vi "RT - Create Or Read Config.vi"(8 "error in":errorcluster) -> (0 "error out":errorcluster)   [LabVIEW 2018]
uses:
  Controls/Config.ctl
  Controls/Settings.ctl
  Controls/Parameters.ctl
  Controls/Timeouts.ctl
  Controls/ConfigString.ctl
  Controls/ConfigData.ctl
  Globals/Global - Configuration Options.vi
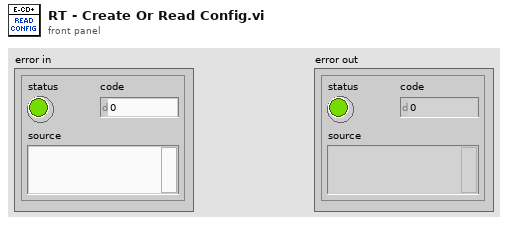
[diagram p1: front panel]
types:
  T1 = typedef "ConfigString.ctl" = cluster{"PDP (IN)":string[], "SETTINGS":string[], "TIMEOUTS (SEC)":string[]}
  T2 = typedef "Timeouts.ctl" = cluster{"TWTT Drive":dbl, "DL Drive":dbl, "DL Rotate":dbl, "BR Drive":dbl, "OT Engage":dbl, "PLUG Drive":dbl, "IT Engage":dbl, "IT 1REV":dbl, "IT nREV":dbl}
  T3 = typedef "Parameters.ctl" = cluster{"PDP (IN)":T4, "SETTINGS":T5, "TIMEOUTS (SEC)":T2}
  T4 = typedef "Config.ctl" = cluster{"TWTT OP":dbl, "TWTT PDP":dbl, "DLT OP":dbl, "DLT PDP 01":dbl, "DLT PDP 02":dbl, "BR OP":dbl, "BR TWT ALIGN":dbl, "BR DL ALIGN":dbl}
  T5 = typedef "Settings.ctl" = cluster{"HPL Low (PSI)":dbl, "HPL High (PSI)":dbl, "HPH Low (PSI)":dbl, "HPH High (PSI)":dbl, "AP Low (PSI)":dbl, "AP High (PSI)":dbl, "DL Clean (SEC)":dbl, "Reset (MIN)":dbl}
  T6 = typedef "ConfigData.ctl" = cluster{"PDP (IN)":dbl[], "SETTINGS":dbl[], "TIMEOUTS (SEC)":dbl[]}
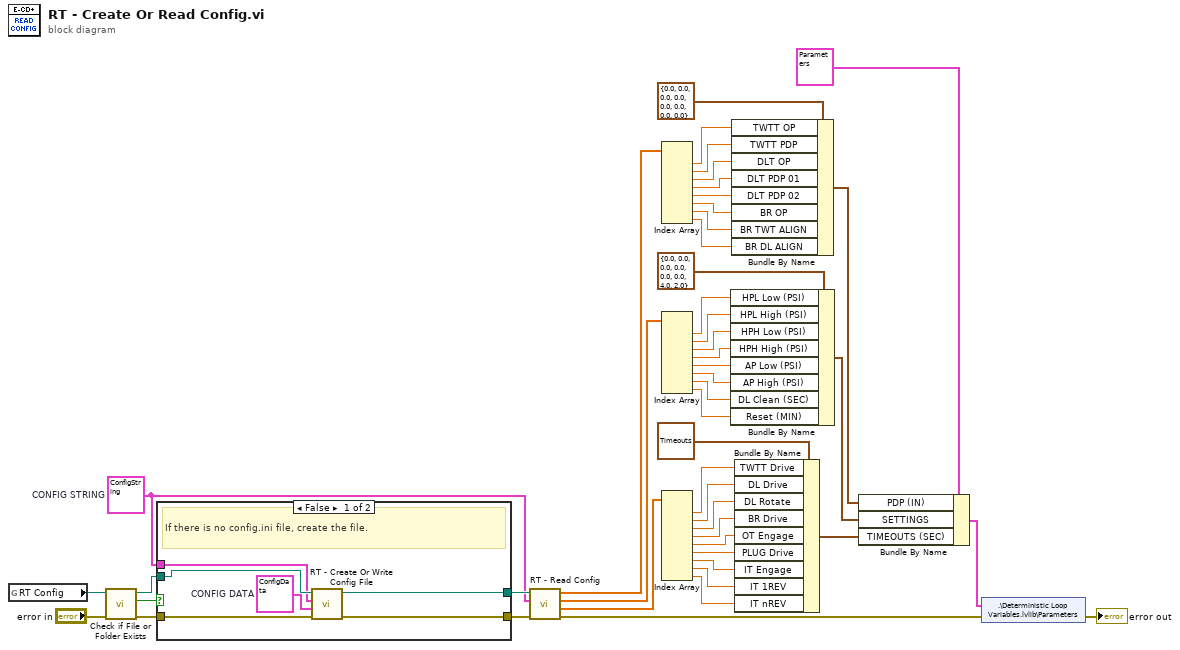
[diagram p0: block diagram]
diagram:
  w31 = T1 {"PDP (IN)"=["TWTT OP (IN)", "TWTT PDP (IN)", "DLT OP (IN)", "DLT PDP 01 (IN)", "DLT PDP 02 (IN)", "BR OP (IN)", "BR TWT ALIGN", "BR DL ALIGN (IN)"], "SETTINGS"=["HPL Low (PSI)", "HPL High (PSI)", "HPH Low (PSI)", "HPH High (PSI)", "AP Low (PSI)", "AP High (PSI)", "DL Clean (SEC)", "Reset (MIN)"], "TIMEOUTS (SEC)"=["TWTT Drive (SEC)", "DL Drive (SEC)", "DL Rotate (SEC)", "BR Drive (SEC)", "OT Engage (SEC)", "Plug Drive (SEC)", "IT Engage (SEC)", "IT 1REV (SEC)", "IT nREV (SEC)"]}  # CONFIG STRING
  n1 = global read "Global - Configuration Options.vi" "RT Config"() -> (w36:path)
  n2 = call <vilib>:"Check if File or Folder Exists.vi"("error in (no error)"="error in", "path"=w36) -> ("error out"=w35:errorcluster, "file or folder exists?"=w37:bool, "dup path"=w34:path)  [unwired: 7 in]
  n3 = case shown="False" w37 {
    tunnel: w35 -> [w52 w53]
    tunnel: w34 -> [w51 w54]
    tunnel: [w50 w53] -> w32
    tunnel: [w49 w54] -> w33
    tunnel: w31 -> [w48 _]
    frame False {
      w47 = T6 {"PDP (IN)"=[1.0, 2.2, 1.0, 1.744, 1.4, 5.3, 0.873, 8.975], "SETTINGS"=[100.0, 500.0, 200.0, 2800.0, 30.0, 180.0, 8.0, 2.0], "TIMEOUTS (SEC)"=[20.0, 20.0, 60.0, 20.0, 20.0, 60.0, 20.0, 30.0, 60.0]}  # CONFIG DATA
      # "If there is no config.ini file, create the file."
      n4 = call "RT - Create Or Write Config File.vi"("error in"=w52, "CONFIG DATA"=w47, "CONFIG STRING"=w48, "ConfigFile Path In"=w51) -> ("error out"=w50:errorcluster, "ConfigFile Path Out"=w49:path)  [unwired: 6 in]
    }
    frame True {
    }
  }
  n5 = call "RT - Read Config.vi"("error in"=w32, "CONFIG STRING"=w31, "ConfigFile Path In"=w33) -> ("error out"=w29:errorcluster, "TIMEOUTS (SEC)"=w15:dbl[], "SETTINGS"=w24:dbl[], "PDP (IN)"=w28:dbl[])  [unwired: 5 in]
  n6 = Index Array(array=w28) -> (element #1=w27:dbl, element #2=w26:dbl, element #3=w25:dbl, element #4=w5:dbl, element #5=w4:dbl, element #6=w3:dbl, element #7=w2:dbl, element #8=w1:dbl)  [unwired: 8 in]
  n7 = Index Array(array=w24) -> (element #1=w23:dbl, element #2=w22:dbl, element #3=w21:dbl, element #4=w20:dbl, element #5=w19:dbl, element #6=w18:dbl, element #7=w17:dbl, element #8=w16:dbl)  [unwired: 8 in]
  n8 = Index Array(array=w15) -> (element #1=w14:dbl, element #2=w13:dbl, element #3=w12:dbl, element #4=w11:dbl, element #5=w10:dbl, element #6=w9:dbl, element #7=w8:dbl, element #8=w7:dbl, element #9=w6:dbl)  [unwired: 9 in]
  n9 = Bundle By Name(cluster=T5 {"HPL Low (PSI)"=0.0, "HPL High (PSI)"=0.0, "HPH Low (PSI)"=0.0, "HPH High (PSI)"=0.0, "AP Low (PSI)"=0.0, "AP High (PSI)"=0.0, "DL Clean (SEC)"=4.0, "Reset (MIN)"=2.0} ("SETTINGS"), "HPL Low (PSI)"=w23, "HPL High (PSI)"=w22, "HPH Low (PSI)"=w21, "HPH High (PSI)"=w20, "AP Low (PSI)"=w19, "AP High (PSI)"=w18, "DL Clean (SEC)"=w17, "Reset (MIN)"=w16) -> (w41:T5)
  n10 = Bundle By Name(cluster=T4 {"TWTT OP"=0.0, "TWTT PDP"=0.0, "DLT OP"=0.0, "DLT PDP 01"=0.0, "DLT PDP 02"=0.0, "BR OP"=0.0, "BR TWT ALIGN"=0.0, "BR DL ALIGN"=0.0} ("Config"), "TWTT OP"=w27, "TWTT PDP"=w26, "DLT OP"=w25, "DLT PDP 01"=w5, "DLT PDP 02"=w4, "BR OP"=w3, "BR TWT ALIGN"=w2, "BR DL ALIGN"=w1) -> (w42:T4)
  n11 = Bundle By Name(cluster=T2 {"TWTT Drive"=20.0, "DL Drive"=20.0, "DL Rotate"=60.0, "BR Drive"=20.0, "OT Engage"=20.0, "PLUG Drive"=60.0, "IT Engage"=20.0, "IT 1REV"=30.0, "IT nREV"=60.0} ("TIMEOUTS"), "TWTT Drive"=w14, "DL Drive"=w13, "DL Rotate"=w12, "BR Drive"=w11, "OT Engage"=w10, "PLUG Drive"=w9, "IT Engage"=w8, "IT 1REV"=w7, "IT nREV"=w6) -> (w38:T2)
  n12 = Bundle By Name(cluster=T3 {"PDP (IN)"={"TWTT OP"=0.0, "TWTT PDP"=0.0, "DLT OP"=0.0, "DLT PDP 01"=0.0, "DLT PDP 02"=0.0, "BR OP"=0.0, "BR TWT ALIGN"=0.0, "BR DL ALIGN"=0.0}, "SETTINGS"={"HPL Low (PSI)"=0.0, "HPL High (PSI)"=0.0, "HPH Low (PSI)"=0.0, "HPH High (PSI)"=0.0, "AP Low (PSI)"=0.0, "AP High (PSI)"=0.0, "DL Clean (SEC)"=4.0, "Reset (MIN)"=2.0}, "TIMEOUTS (SEC)"={"TWTT Drive"=20.0, "DL Drive"=20.0, "DL Rotate"=60.0, "BR Drive"=20.0, "OT Engage"=20.0, "PLUG Drive"=60.0, "IT Engage"=20.0, "IT 1REV"=30.0, "IT nREV"=60.0}} ("PARAMETERS"), "PDP (IN)"=w42, "SETTINGS"=w41, "TIMEOUTS (SEC)"=w38) -> (w40:T3)
  n13 = shared-variable ".\\Deterministic Loop Variables.lvlib\\Parameters"(w40, error in=w29) -> (error out=→"error out":errorcluster)
